vi "ReceiveMotorData.vi"(4 "Timeout ms":i32=1, 6 "Positions":dbl[](array[numeric]), 7 "MotorData Input":T1(array[cluster]), 8 "Override Data":bool, 9 "UDP Input":T2) -> (0 "Error Out":errorcluster, 1 "MotorData Output":T1(array[cluster]), 2 "Valid Data":bool, 3 "UDP Output":T2)   [LabVIEW 2019]
panel:
  out "New Force Instruction":bool[](array[boolean])=[TRUE, TRUE, TRUE]
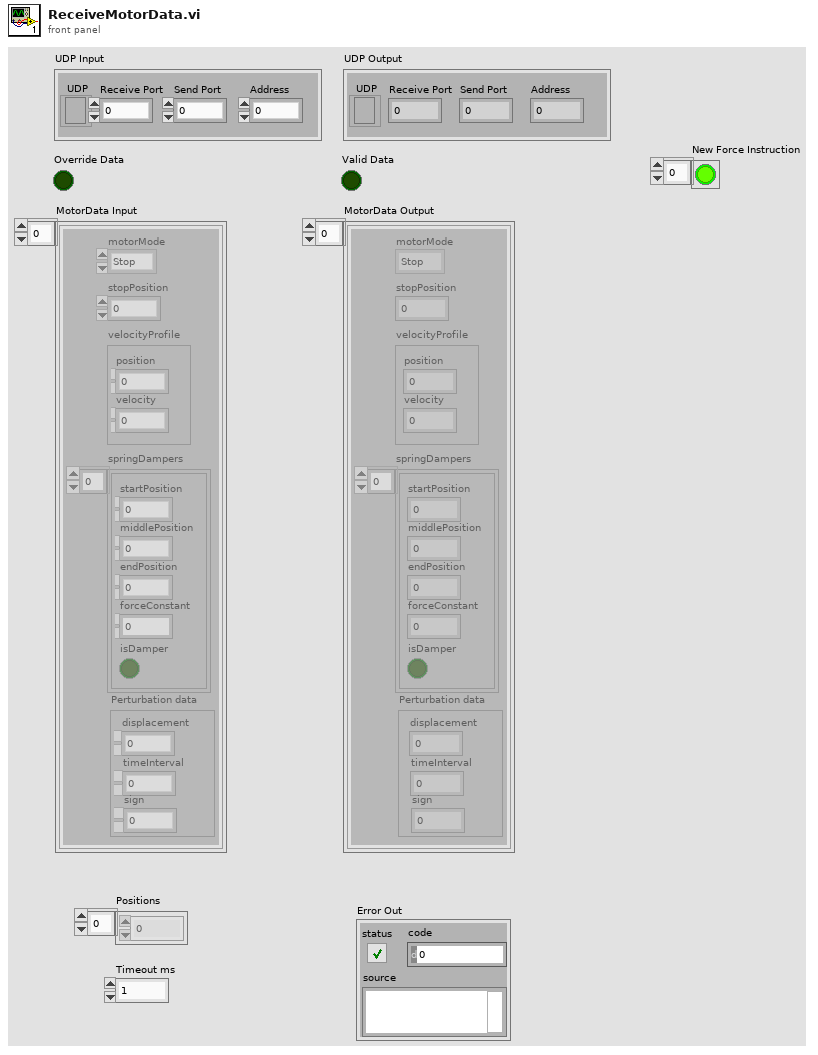
[diagram p1: front panel]
types:
  T1 = cluster{"motorMode":enum16{"Stop", "Move", "Force", "Perturbation"}, "stopPosition":dbl, "velocityProfile":cluster{"position":dbl, "velocity":dbl}, "springDampers":cluster{"startPosition":dbl, "middlePosition":dbl, "endPosition":dbl, "forceConstant":dbl, "isDamper":bool}[], "Perturbation data ":cluster{"displacement":dbl, "timeInterval":dbl, "sign":i64}}[]
  T2 = cluster{"UDP":refnum<k16>, "Receive Port":i32, "Send Port":i32, "Address":i64}
  T3 = cluster{"motorMode":enum16{"Stop", "Move", "Force", "Perturbation"}, "stopPosition":dbl, "velocityProfile":cluster{"position":dbl, "velocity":dbl}, "springDampers":cluster{"startPosition":dbl, "middlePosition":dbl, "endPosition":dbl, "forceConstant":dbl, "isDamper":bool}[], "Perturbation data ":cluster{"displacement":dbl, "timeInterval":dbl, "sign":i64}}
  T4 = cluster{"motor":i8, "mode":i8, "jsonData":string}
  T5 = cluster{"startPosition":dbl, "middlePosition":dbl, "endPosition":dbl, "forceConstant":dbl, "isDamper":bool}[]
  T6 = cluster{"startPosition":dbl, "middlePosition":dbl, "endPosition":dbl, "forceConstant":dbl, "isDamper":bool}
  T7 = cluster{"displacement":dbl, "timeInterval":dbl, "sign":i64}
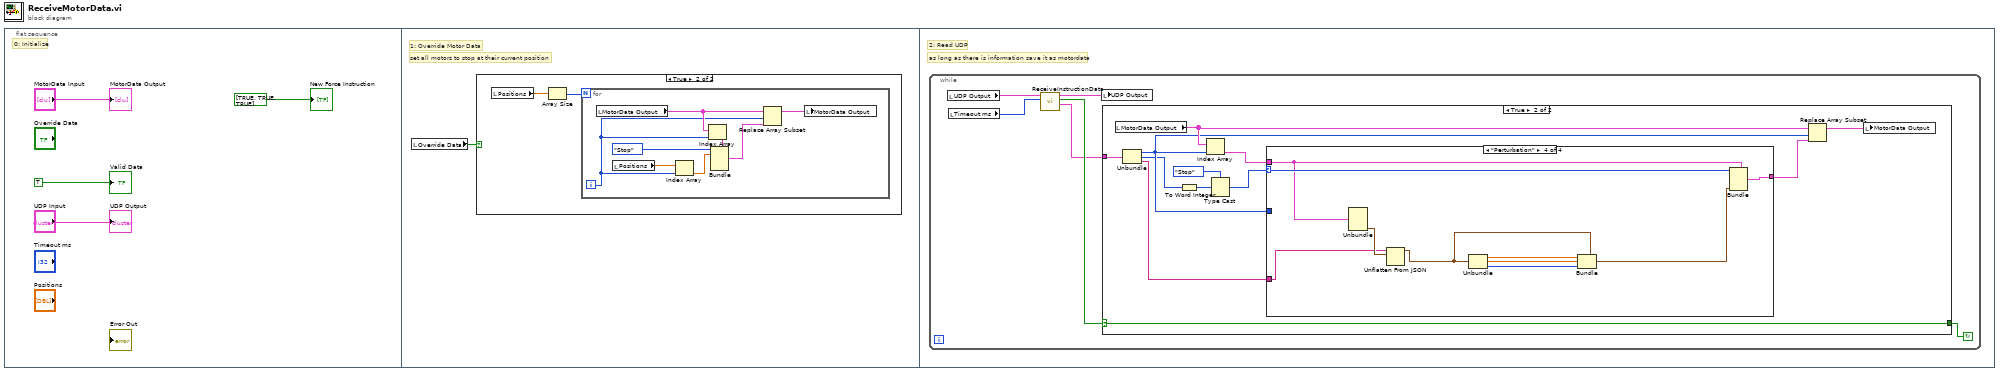
[diagram p0: block diagram]
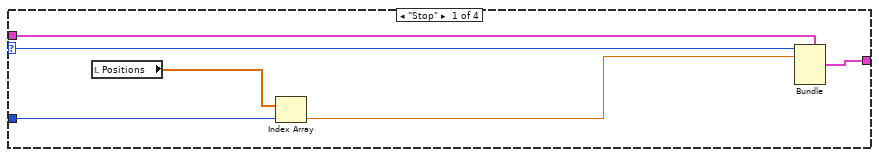
[diagram p4: hidden frame]
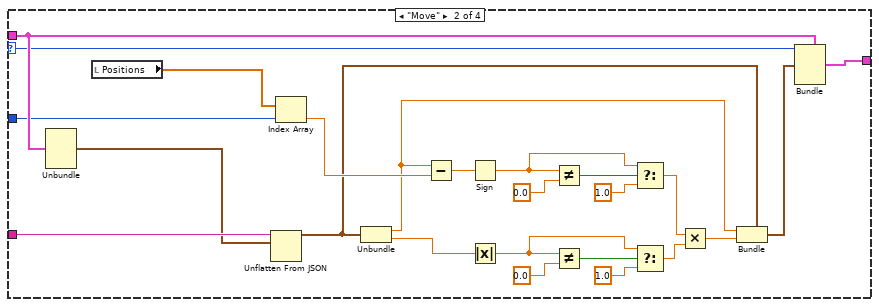
[diagram p5: hidden frame]
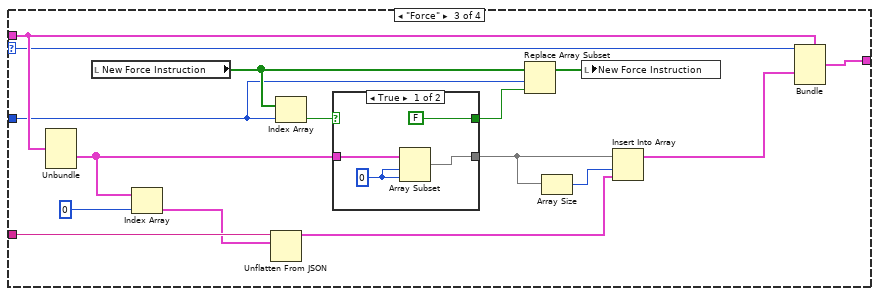
[diagram p6: hidden frame]
diagram:
  n1 = flat-sequence {
    frame #0 {
      # "0: Initialize"
      "Valid Data" <- TRUE
      "UDP Output" <- "UDP Input"
      "New Force Instruction" <- bool[] [TRUE, TRUE, TRUE] ("New Force Instruction")
      "MotorData Output" <- "MotorData Input"
    }
    frame #1 {
      # "set all motors to stop at their current position"
      # "1: Override Motor Data"
      n2 = local read "Override Data"() -> (w5:bool)
      n3 = case shown="True" w5 {
        frame False {
        }
        frame True {
          n4 = local read "Positions"() -> (w6:dbl[])
          n5 = Array Size(array=w6) -> (size(s)=w7:i32)
          n6 = for {
            N: w7 -> [_]
            i -> [w9]
            n7 = local read "MotorData Output"() -> (w11:T1)
            n8 = local read "Positions"() -> (w13:dbl[])
            n9 = Index Array(array=w13, index=w9) -> (element=w12:dbl)
            n10 = Index Array(array=w11, index=w9) -> (element=w14:T3)
            n11 = Bundle(cluster=w14, "motorMode"=enum16{"Stop", "Move", "Force", "Perturbation"}."Stop" ("MotorMode"), "stopPosition"=w12) -> (w10:T3)  [unwired: 3 in]
            n12 = Replace Array Subset(array=w11, new element=w10, index=w9) -> (w8:T1)
            n13 = local write "MotorData Output"(w8) -> ()
          }
        }
      }
    }
    frame #2 {
      # "as long as there is information save it as motordata"
      # "2: Read UDP"
      n14 = while {
        stop <- w21 continue-if-true
        n15 = local read "UDP Output"() -> (w20:T2)
        n16 = local read "Timeout ms"() -> (w18:i32)
        n17 = call "ReceiveInstructionData.vi"("Timeout ms"=w18, "UDP Input"=w20) -> ("MotorInstuction Output"=w16:T4, "Did Receive"=w17:bool, "UDP Output"=w19:T2)  [unwired: 2 in, 1 out]
        n18 = local write "UDP Output"(w19) -> ()
        n19 = case shown="True" w17 {
          selector: w17 -> [w22 w34]
          tunnel: [w22 w34] -> w21
          tunnel: w16 -> [_ w33]
          frame False {
          }
          frame True {
            n20 = local read "MotorData Output"() -> (w31:T1)
            n21 = Unbundle(w33) -> ("motor"=w25:i8, "mode"=w23:i8, "jsonData"=w27:string)
            n22 = To Word Integer(number=w23) -> (16bit integer=w24:i16)
            n23 = Index Array(array=w31, index=w25) -> (element=w28:T3)
            n24 = Type Cast(type=enum16{"Stop", "Move", "Force", "Perturbation"}."Stop" ("MotorMode"), x=w24) -> (*(type *) &x=w29:enum16{"Stop", "Move", "Force", "Perturbation"})
            n25 = case shown="\"Perturbation\"" w29 {
              selector: w29 -> [w38 w61 w65 w95]
              tunnel: w28 -> [w39 w63 w79 w94]
              tunnel: w27 -> [_ w62 w71 w91]
              tunnel: [w40 w64 w80 w96] -> w26
              tunnel: w25 -> [w36 w58 w73 _]
              frame "Stop" {
                n26 = local read "Positions"() -> (w37:dbl[])
                n27 = Index Array(array=w37, index=w36) -> (element=w35:dbl)
                n28 = Bundle(cluster=w39, "motorMode"=w38, "stopPosition"=w35) -> (w40:T3)  [unwired: 3 in]
              }
              frame "Move" {
                n29 = Unbundle(w63) -> ("velocityProfile"=w60:cluster{"position":dbl, "velocity":dbl})  [unwired: 4 out]
                n30 = local read "Positions"() -> (w59:dbl[])
                n31 = Unflatten From JSON(JSON string=w62, type and defaults=w60) -> (value=w43:cluster{"position":dbl, "velocity":dbl})  [unwired: 5 in, 1 out]
                n32 = Index Array(array=w59, index=w58) -> (element=w57:dbl)
                n33 = Unbundle(w43) -> ("position"=w42:dbl, "velocity"=w51:dbl)
                n34 = Subtract(x=w42, y=w57) -> (x-y=w56:dbl)
                n35 = Sign(1:w56) -> (0:w53:dbl)
                n36 = Absolute Value(x=w51) -> (abs(x)=w45:dbl)
                n37 = Not Equal?(x=w53, y=0.0) -> (x != y?=w54:bool)
                n38 = Not Equal?(x=w45, y=0.0) -> (x != y?=w48:bool)
                n39 = Select(t=w53, s=w54, f=1.0) -> (s? t:f=w50:dbl)
                n40 = Select(t=w45, s=w48, f=1.0) -> (s? t:f=w46:dbl)
                n41 = Multiply(x=w50, y=w46) -> (x*y=w41:dbl)
                n42 = Bundle(cluster=w43, "position"=w42, "velocity"=w41) -> (w44:cluster{"position":dbl, "velocity":dbl})
                n43 = Bundle(cluster=w63, "motorMode"=w61, "velocityProfile"=w44) -> (w64:T3)  [unwired: 3 in]
              }
              frame "Force" {
                n44 = Unbundle(w79) -> ("springDampers"=w69:T5)  [unwired: 4 out]
                n45 = local read "New Force Instruction"() -> (w75:bool[])
                n46 = Index Array(array=w69, index=0) -> (element=w68:T6)
                n47 = Unflatten From JSON(JSON string=w71, type and defaults=w68) -> (value=w67:T6)  [unwired: 5 in, 1 out]
                n48 = Index Array(array=w75, index=w73) -> (element=w76:bool)
                n49 = case shown="True" w76 {
                  selector: w76 -> [_ w85]
                  tunnel: [FALSE w85] -> w77
                  tunnel: w69 -> [w83 w86]
                  tunnel: [w82 w86] -> w72
                  frame True {
                    w84 = 0
                    n50 = Array Subset(array=w83, index=w84, length=w84) -> (w82:T5)
                  }
                  frame False {
                  }
                }
                n51 = Replace Array Subset(array=w75, new element=w77, index=w73) -> (w74:bool[])
                n52 = Array Size(array=w72) -> (size(s)=w78:i32)
                n53 = local write "New Force Instruction"(w74) -> ()
                n54 = Insert Into Array(array=w72, index=w78, new element=w67) -> (w66:T5)
                n55 = Bundle(cluster=w79, "motorMode"=w65, "springDampers"=w66) -> (w80:T3)  [unwired: 3 in]
              }
              frame "Perturbation" {
                n56 = Unbundle(w94) -> ("Perturbation data"=w93:T7)  [unwired: 4 out]
                n57 = Unflatten From JSON(JSON string=w91, type and defaults=w93) -> (value=w90:T7)  [unwired: 5 in, 1 out]
                n58 = Unbundle(w90) -> ("displacement"=w87:dbl, "timeInterval"=w88:dbl, "sign"=w89:i64)
                n59 = Bundle(cluster=w90, "displacement"=w87, "timeInterval"=w88, "sign"=w89) -> (w92:T7)
                n60 = Bundle(cluster=w94, "motorMode"=w95, "Perturbation data"=w92) -> (w96:T3)  [unwired: 3 in]
              }
            }
            n61 = Replace Array Subset(array=w31, new element=w26, index=w25) -> (w32:T1)
            n62 = local write "MotorData Output"(w32) -> ()
          }
        }
      }
    }
  }
